vi "Abort Motion.vi"(8 "error in (no error)":errorcluster, 11 "Gantry in":refnum<class "A3200.lvclass">) -> (0 "error out":errorcluster, 3 "Gantry out":refnum<class "A3200.lvclass">)   [LabVIEW 2016, in "A3200.lvclass"]
uses:
  A3200.lvclass
  A3200.lvclass/A3200.ctl
  <userlib>/Aerotech A3200.lnk/Aerotech VIs.lvlib
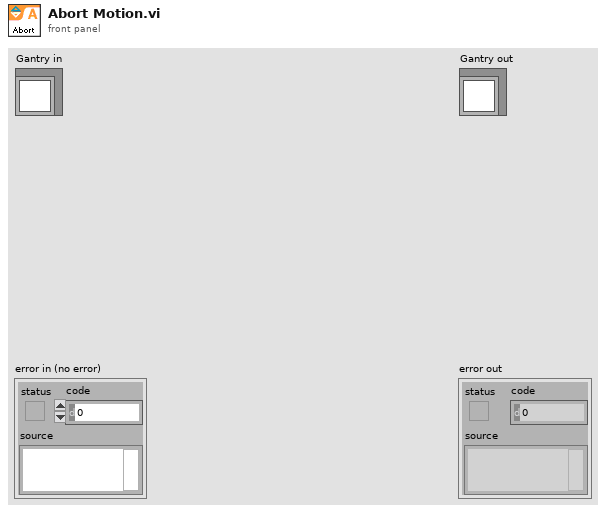
[diagram p1: front panel]
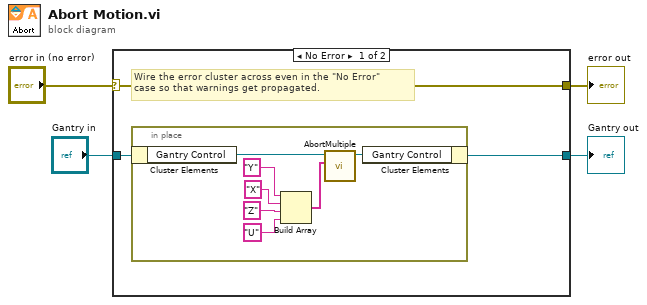
[diagram p0: block diagram]
diagram:
  n1 = case shown="No Error" "error in (no error)" {
    selector: "error in (no error)" -> [w7 w16]
    tunnel: [w7 w16] -> w3
    tunnel: [w5 w15] -> w1
    tunnel: "Gantry in" -> [w6 w15]
    frame No Error {
      # "Wire the error cluster across even in the \"No Error\"\ncase so that warnings get propagated."
      n2 = in-place {
        n3 = in-place-cluster #1(w6) -> ("Gantry Control"=w9:refnum<k24>)
        n4 = Build Array("Y", "X", "Z", "U") -> (w10:string[])
        n5 = call <userlib>:"AbortMultiple.vi"("axis names"=w10, "controller in"=w9) -> ("controller out"=w8:refnum<k24>)  [unwired: 8 in, 1 out]
        n6 = in-place-cluster #1("Gantry Control"=w8) -> (w5:refnum<class "A3200.lvclass">)
      }
    }
    frame Error {
    }
  }
  "error out" <- w3
  "Gantry out" <- w1
